vi "Split file name.vi"(11 "file name":string="^[0-9]+") -> (2 "extension":string="^[0-9]+", 3 "name":string="^[0-9]+", 4 "exact match":bool)   [LabVIEW 2015]
uses:
  <vilib>/regexp/Match Regular Expression.xnode
panel:
  in  "regular expression":string="^[0-9]+"
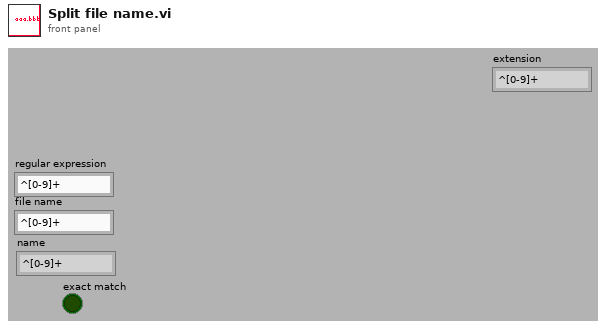
[diagram p1: front panel]
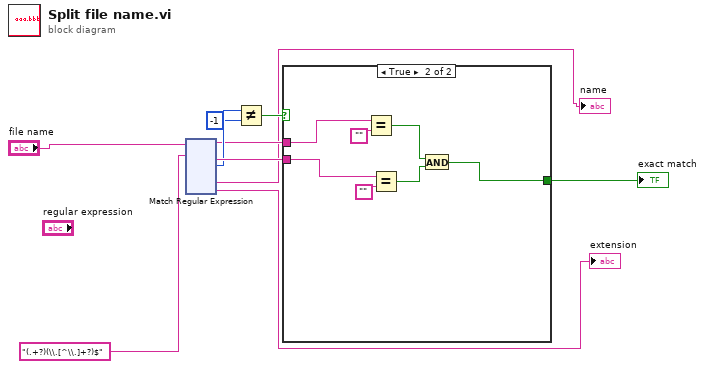
[diagram p0: block diagram]
diagram:
  n1 = xnode "Match Regular Expression"("input string"="file name", "regular expression"="(.+?)(\\.[^\\.]+?)$" ("string")) -> ("before match"=w7:string, "after match"=w10:string, "offset past match"=w9:i32, "submatch 1"=→"name":string, "submatch 2"=→"extension":string)  [unwired: 4 in, 2 out]
  n2 = Not Equal?(x=w9, y=-1) -> (x != y?=w6:bool)
  n3 = case shown="True" w6 {
    selector: w6 -> [w11 _]
    tunnel: w10 -> [_ w17]
    tunnel: w7 -> [_ w12]
    tunnel: [w11 w13] -> w5
    frame False {
    }
    frame True {
      n4 = Equal?(x=w12, y="") -> (x = y?=w14:bool)
      n5 = Equal?(x=w17, y="") -> (x = y?=w15:bool)
      n6 = And(x=w14, y=w15) -> (x .and. y?=w13:bool)
    }
  }
  "exact match" <- w5
